vi "Time.Day Index from Start.vi"(10 "Test Time":timestamp, 11 "Start Day":timestamp) -> (3 "Index":i32)   [LabVIEW 2019]
uses:
  Time.DateTime Adjust Action.ctl
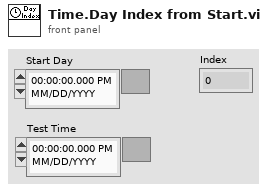
[diagram p1: front panel]
types:
  T1 = typedef "Time.DateTime Adjust Action.ctl" = enum16{"Day Start", "Day End", "Offset Hrs", "UTC to Local", "Local to UTC"}
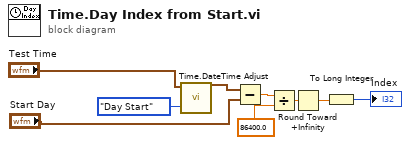
[diagram p0: block diagram]
diagram:
  n1 = call "Time.DateTime Adjust.vi"("Action"=Time.DateTime_Adjust_Action."Day Start", "Time Stamp"="Test Time") -> ("Time Stamp Out"=w4:timestamp)  [unwired: 8 in, 1 out]
  n2 = Subtract(x=w4, y="Start Day") -> (x-y=w5:dbl)
  n3 = Divide(x=w5, y=86400.0) -> (x/y=w7:dbl)
  n4 = Round Toward +Infinity(x=w7) -> (ceil(x): smallest int >= x=w8:dbl)
  n5 = To Long Integer(number=w8) -> (32bit integer=→"Index":i32)
